vi "Init_Device.vi"(8 "error in (no error)":errorcluster, 10 "Baud Rate (115200)":u32=115200, 11 "COM Port":refnum<visa-resource-name>="COM1") -> (0 "error out":errorcluster, 3 "Device":T1)   [LabVIEW 2017]
uses:
  device.ctl
  <vilib>/Instr/_visa.llb/VISA Configure Serial Port (Instr).vi
panel:
  in  "Sample rate (1 ms)":u32=1
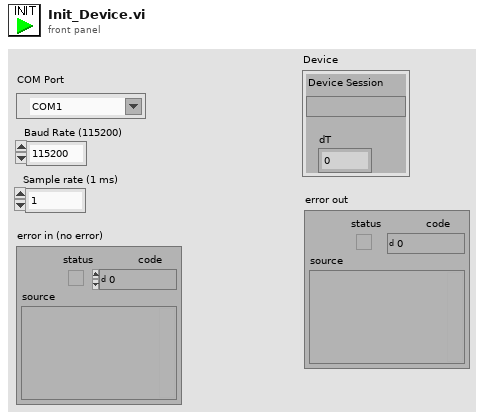
[diagram p1: front panel]
types:
  T1 = typedef "device.ctl" = cluster{"Device Session":refnum<visa-resource-name>, "dT":i32}
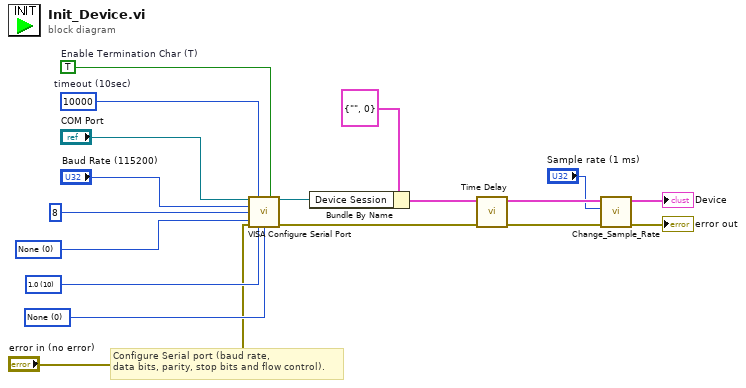
[diagram p0: block diagram]
diagram:
  w10 = u16 0 items=["None"=0, "XON/XOFF"=1, "RTS/CTS"=2, "DTR/DSR"=4] ("flow control")
  w11 = u16 10 items=["1.0"=10, "1.5"=15, "2.0"=20] ("stop bits")
  w14 = u16 0 items=["None", "Odd", "Even", "Mark", "Space"] ("parity")
  w12 = TRUE  # Enable Termination Char (T)
  w13 = u32 10000  # timeout (10sec)
  # "Configure Serial port (baud rate,\ndata bits, parity, stop bits and flow control)."
  n1 = call-poly "VISA Configure Serial Port"("VISA resource name"="COM Port", "timeout (10sec)"=w13, "Enable Termination\nChar (T)"=w12, "baud rate (9600)"="Baud Rate (115200)", "data bits (8)"=u16 8 ("data bits"), "parity (0:none)"=w14, "error in (no error)"="error in (no error)", "stop bits (10: 1 bit)"=w11, "flow control (0:none)"=w10) -> ("VISA resource name out"=w8:refnum<visa-resource-name>, "error out"=w4:errorcluster)  [unwired: 5 in]
  n2 = Bundle By Name(cluster=T1 {"Device Session"="", "dT"=0} ("Device"), "Device Session"=w8) -> (w17:T1)
  n3 = call "Time Delay"("error in (no error)"=w4) -> ("error out"=w3:errorcluster)  [unwired: 10 in]
  n4 = call "Change_Sample_Rate.vi"("error in"=w3, "Period [ms]"="Sample rate (1 ms)", "Device IN"=w17) -> ("error out"=→"error out":errorcluster, "Device OUT"=→"Device":T1)  [unwired: 7 in]
